vi "Delete Icon Editor from LV Installation.vi"(8 "error in":errorcluster) -> (0 "error out":errorcluster, 3 "were files previously present?":bool)   [LabVIEW 2021]
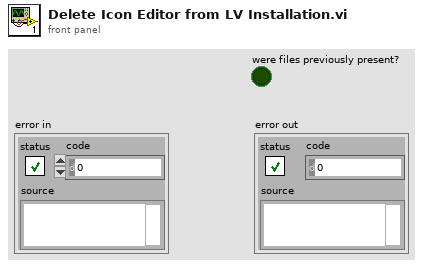
[diagram p1: front panel]
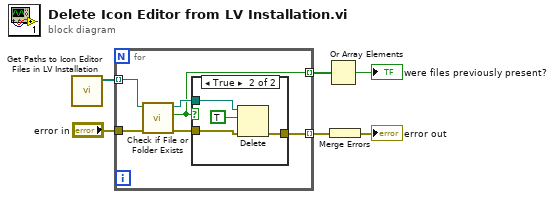
[diagram p0: block diagram]
diagram:
  n1 = call <resource>:"Get Paths to Icon Editor Files in LV Installation.vi"() -> ("paths"=w3:path[])  [unwired: 11 in]
  n2 = for {
    tunnel: w3 -> [w11] mode=indexing
    tunnel: "error in" -> [w10]
    tunnel: [w12] -> w4 mode=indexing
    tunnel: [w7] -> w2 mode=indexing
    n3 = call <vilib>:"Check if File or Folder Exists.vi"("error in (no error)"=w10, "path"=w11) -> ("error out"=w9:errorcluster, "file or folder exists?"=w7:bool, "dup path"=w8:path)  [unwired: 7 in]
    n4 = case shown="True" w7 {
      tunnel: w9 -> [w13 w17]
      tunnel: [w13 w16] -> w12
      tunnel: w8 -> [_ w14]
      frame False {
      }
      frame True {
        n5 = Delete(path (use dialog)=w14, entire hierarchy (F)=TRUE, error in=w17) -> (error out=w16:errorcluster)  [unwired: 2 in, 2 out]
      }
    }
  }
  n6 = Or Array Elements(Boolean array=w2) -> (logical OR=→"were files previously present?":bool)
  n7 = Merge Errors(w4) -> (→"error out":errorcluster)
